vi "WriteBase.vi"(0 "GenericCanAdapterClass in":refnum<class "GenericCanAdapterClass.lvclass">, 5 "Id":u32 format="%08x", 7 "DataLength":i32, 9 "Data":u8[](array[numeric]) format="%02x", 11 "error in (no error)":errorcluster) -> (4 "GenericCanAdapterClass out":refnum<class "GenericCanAdapterClass.lvclass">, 15 "error out":errorcluster)   [LabVIEW 2011, in "GenericCanAdapterClass.lvclass"]
uses:
  GenericCanAdapterClass.lvclass
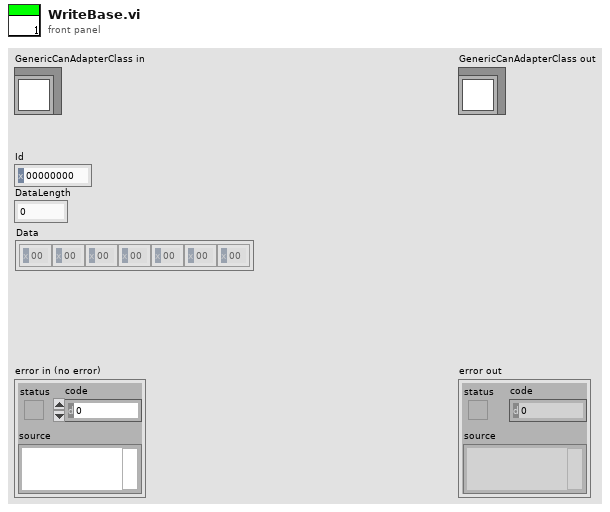
[diagram p1: front panel]
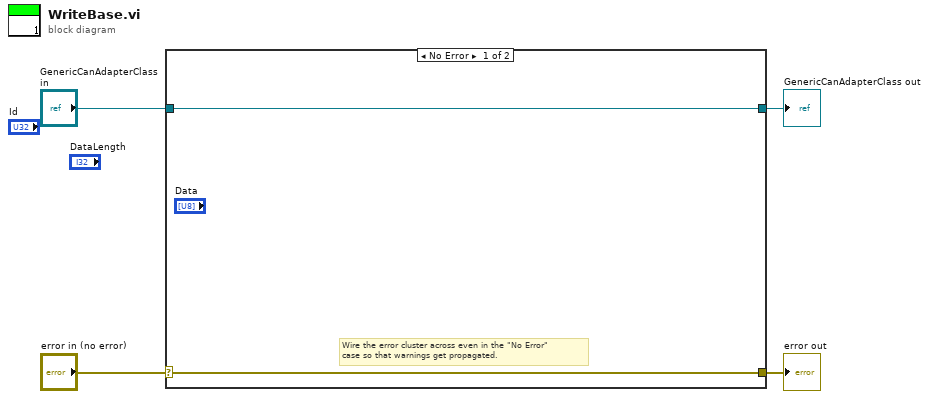
[diagram p0: block diagram]
diagram:
  n1 = case shown="No Error" "error in (no error)" {
    selector: "error in (no error)" -> [w5 w8]
    tunnel: [w5 w8] -> w3
    tunnel: [w6 w7] -> w1
    tunnel: "GenericCanAdapterClass in" -> [w6 w7]
    frame No Error {
      # "Wire the error cluster across even in the \"No Error\"\ncase so that warnings get propagated."
    }
    frame Error {
    }
  }
  "error out" <- w3
  "GenericCanAdapterClass out" <- w1
